vi "dV(dRo)Arch.vi"() -> ()   [LabVIEW 2023]
panel:
  out "x > y?":bool
  out "L см":dbl format="%#_3f"
  out "v м3":dbl format="%#_3f"
  out "Enum":enum16{"ХОВ", "Бор"}(ring)
  in  "dRo":dbl
  in  "N ГЦП":dbl
  in  "C подпитка":dbl
  in  "C крайно":dbl
  in  "C начално":dbl
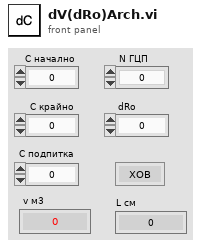
[diagram p1: front panel]
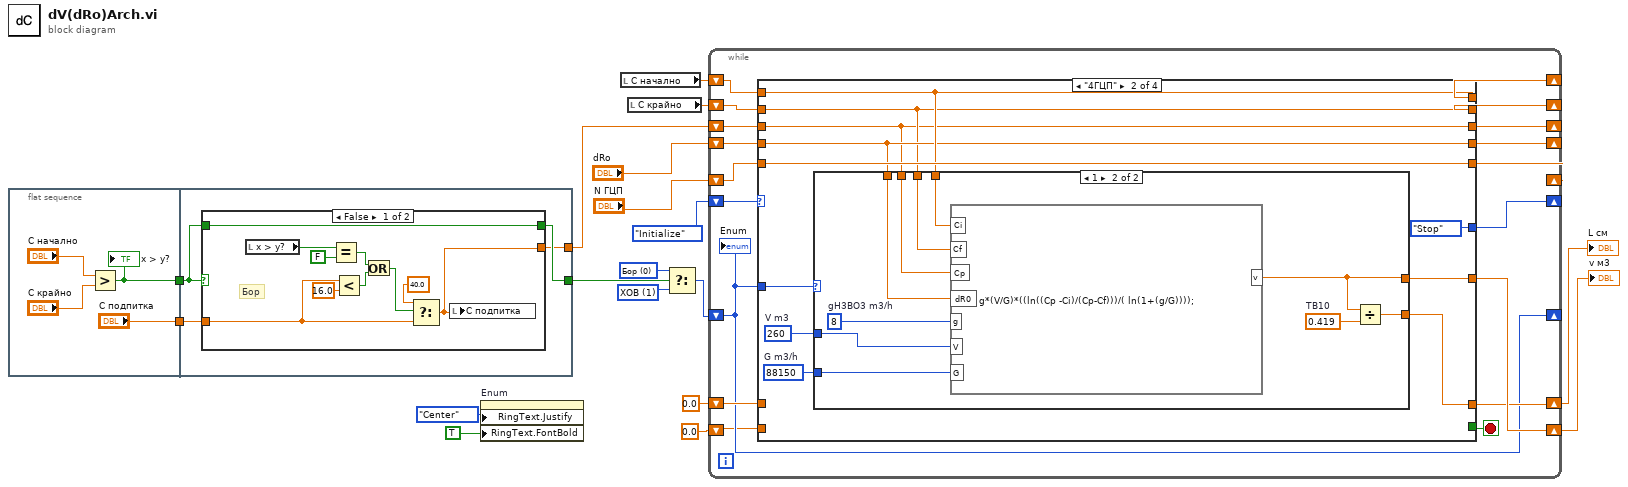
[diagram p0: block diagram]
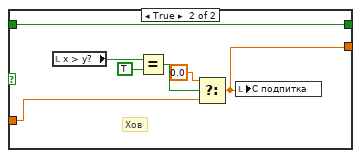
[diagram p2: hidden frame]
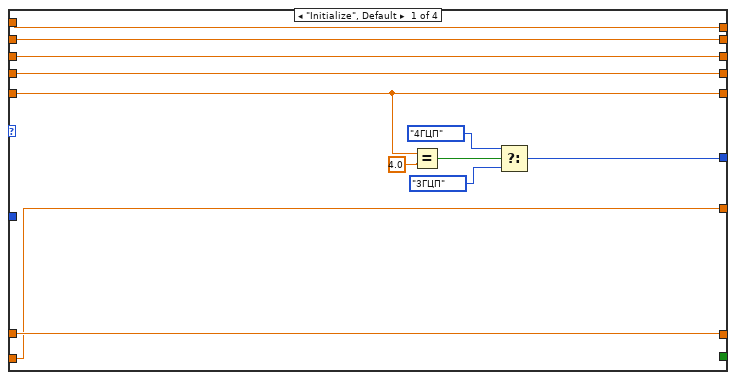
[diagram p3: hidden frame]
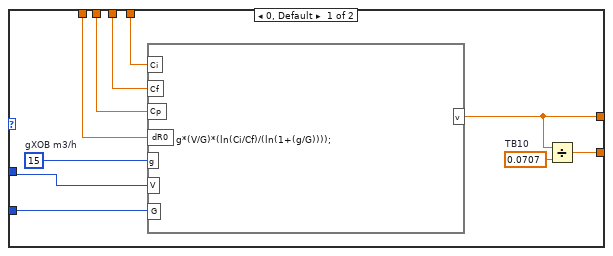
[diagram p4: hidden frame]
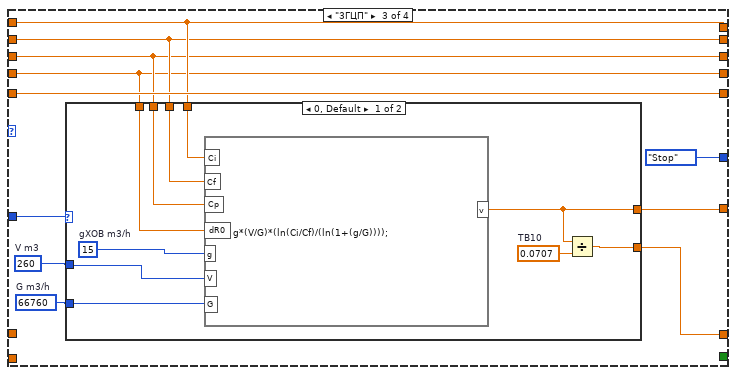
[diagram p5: hidden frame]
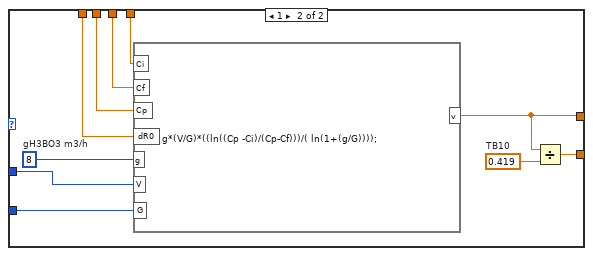
[diagram p6: hidden frame]
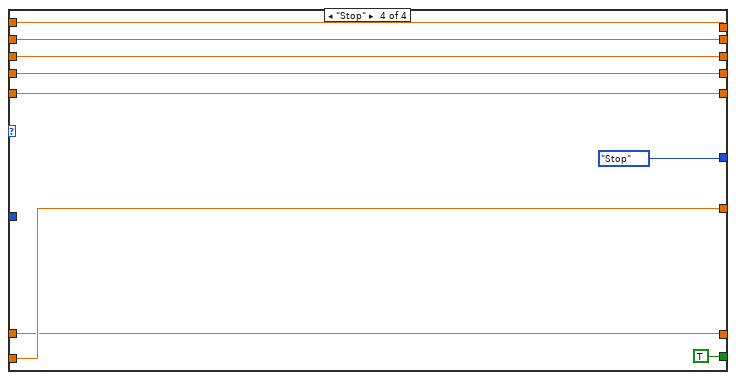
[diagram p7: hidden frame]
diagram:
  w12 = u16 0 items=["Бор", "ХОВ"]
  w13 = u16 1 items=["Бор", "ХОВ"]
  n1 = flat-sequence {
    tunnel: [w22] -> w7
    tunnel: ["C подпитка"] -> w5
    tunnel: [w25] -> w8
    tunnel: w7 -> [w26]
    tunnel: [w24] -> w6
    tunnel: w5 -> [w23]
    frame #0 {
      n2 = Greater?(x="C начално", y="C крайно") -> (0:w22:bool)
      "x > y?" <- w22
    }
    frame #1 {
      n3 = case shown="False" w26 {
        tunnel: w26 -> [w29 w43]
        tunnel: [w29 w43] -> w25
        tunnel: [w28 w37] -> w24
        tunnel: w23 -> [w27 w38]
        frame False {
          # "Бор"
          n4 = local read "x > y?"() -> (w33:bool)
          n5 = Equal?(x=w33, y=FALSE) -> (x = y?=w35:bool)
          n6 = Less?(x=w27, y=16.0) -> (x < y?=w34:bool)
          n7 = Or(x=w35, y=w34) -> (x .or. y?=w36:bool)
          n8 = Select(t=40.0, s=w36, f=w27) -> (s? t:f=w28:dbl)
          n9 = local write "C подпитка"(w28) -> ()
        }
        frame True {
          # "Хов"
          n10 = local read "x > y?"() -> (w41:bool)
          n11 = Equal?(x=w41, y=TRUE) -> (x = y?=w42:bool)
          n12 = Select(t=0.0, s=w42, f=w38) -> (s? t:f=w37:dbl)
          n13 = local write "C подпитка"(w37) -> ()
        }
      }
    }
  }
  n14 = property on="Enum" class="Enum (strict)"("RingText.Justify"=enum16{"Left", "Center", "Right"}."Center" ("Ring Text.Justification"), "RingText.FontBold"=TRUE ("Ring Text.Font:Bold")) -> ()  [unwired: 2 in, 2 out]
  n15 = local read "C начално"() -> (w4:dbl)
  n16 = local read "C крайно"() -> (w3:dbl)
  n17 = Select(t=w12, s=w8, f=w13) -> (s? t:f=w14:u16)
  n18 = while {
    shift-right: [w59] -> _
    shift-left: w4 -> [w60]
    shift-right: [w57] -> _
    shift-left: w3 -> [w58]
    shift-right: [w55] -> _
    shift-left: w6 -> [w56]
    shift-right: [w53] -> _
    shift-left: "dRo" -> [w54]
    shift-right: [w50] -> _
    shift-left: enum16{"Initialize", "4ГЦП", "3ГЦП", "Stop"}."Initialize" -> [w61]
    shift-right: [w51] -> _
    shift-left: "N ГЦП" -> [w52]
    shift-right: [w47] -> w9
    shift-left: 0.0 ("v") -> [w46]
    shift-right: [w45] -> _
    shift-left: w14 -> [w45]
    shift-right: [w48] -> w11
    shift-left: 0.0 ("v") -> [w44]
    stop <- w49 stop-if-true
    n19 = case shown="\"4ГЦП\"" w61 {
      tunnel: w60 -> [w73 w81 w114 w143]
      tunnel: [w73 w81 w114 w143] -> w59
      tunnel: w58 -> [w72 w79 w113 w142]
      tunnel: [w72 w79 w113 w142] -> w57
      tunnel: w56 -> [w71 w78 w112 w141]
      tunnel: [w71 w78 w112 w141] -> w55
      tunnel: w54 -> [w62 w80 w111 w140]
      tunnel: [w62 w80 w111 w140] -> w53
      tunnel: w52 -> [w70 w82 w115 w144]
      tunnel: [w70 w82 w115 w144] -> w51
      tunnel: [w65 enum16{"Initialize", "4ГЦП", "3ГЦП", "Stop"}."Stop" enum16{"Initialize", "4ГЦП", "3ГЦП", "Stop"}."Stop" enum16{"Initialize", "4ГЦП", "3ГЦП", "Stop"}."Stop"] -> w50
      tunnel: [w63 w75 w106 w137] -> w48
      tunnel: [_ _ _ TRUE] -> w49
      tunnel: [w64 w74 w105 w136] -> w47
      tunnel: w46 -> [w64 _ _ w136]
      tunnel: w45 -> [_ w76 w107 _]
      tunnel: w44 -> [w63 _ _ w137]
      frame "Initialize", Default {
        n20 = Equal?(x=w70, y=4.0) -> (x = y?=w68:bool)
        n21 = Select(t=enum16{"Initialize", "4ГЦП", "3ГЦП"}."4ГЦП", s=w68, f=enum16{"Initialize", "4ГЦП", "3ГЦП"}."3ГЦП") -> (s? t:f=w65:enum16{"Initialize", "4ГЦП", "3ГЦП"})
      }
      frame "4ГЦП" {
        w83 = 88150  # G m3/h
        w84 = 260  # V m3
        n22 = case shown="1" w76 {
          tunnel: w84 -> [w93 w101]
          tunnel: w83 -> [w94 w102]
          tunnel: w80 -> [w91 w103]
          tunnel: w78 -> [w90 w96]
          tunnel: w79 -> [w89 w104]
          tunnel: w81 -> [w88 w95]
          tunnel: [w86 w98] -> w75
          tunnel: [w85 w97] -> w74
          frame 0, Default {
            w87 = 0.0707  # TB10
            w92 = 15  # gХОВ m3/h
            n23 = formula code="v = g*(V/G)*(ln(Ci/Cf)/(ln(1+(g/G))));"("Ci"=w88, "Cf"=w89, "Cp"=w90, "dR0"=w91, "g"=w92, "V"=w93, "G"=w94) -> ("v"=w86:dbl)
            n24 = Divide(x=w86, y=w87) -> (x/y=w85:dbl)
          }
          frame 1 {
            w99 = 0.419  # TB10
            w100 = 8  # gH3BO3 m3/h
            n25 = formula code="v = g*(V/G)*((ln((Cp -Ci)/(Cp-Cf)))/( ln(1+(g/G))));"("Ci"=w95, "Cf"=w104, "Cp"=w96, "dR0"=w103, "g"=w100, "V"=w101, "G"=w102) -> ("v"=w98:dbl)
            n26 = Divide(x=w98, y=w99) -> (x/y=w97:dbl)
          }
        }
      }
      frame "3ГЦП" {
        w110 = 66760  # G m3/h
        w109 = 260  # V m3
        n27 = case shown="0, Default" w107 {
          tunnel: w109 -> [w124 w130]
          tunnel: w110 -> [w125 w131]
          tunnel: w111 -> [w122 w132]
          tunnel: w112 -> [w121 w133]
          tunnel: w113 -> [w120 w134]
          tunnel: w114 -> [w119 w135]
          tunnel: [w117 w126] -> w106
          tunnel: [w116 w127] -> w105
          frame 0, Default {
            w118 = 0.0707  # TB10
            w123 = 15  # gХОВ m3/h
            n28 = formula code="v = g*(V/G)*(ln(Ci/Cf)/(ln(1+(g/G))));"("Ci"=w119, "Cf"=w120, "Cp"=w121, "dR0"=w122, "g"=w123, "V"=w124, "G"=w125) -> ("v"=w117:dbl)
            n29 = Divide(x=w117, y=w118) -> (x/y=w116:dbl)
          }
          frame 1 {
            w128 = 0.419  # TB10
            w129 = 8  # gH3BO3 m3/h
            n30 = formula code="v = g*(V/G)*((ln((Cp -Ci)/(Cp-Cf)))/( ln(1+(g/G))));"("Ci"=w135, "Cf"=w134, "Cp"=w133, "dR0"=w132, "g"=w129, "V"=w130, "G"=w131) -> ("v"=w126:dbl)
            n31 = Divide(x=w126, y=w128) -> (x/y=w127:dbl)
          }
        }
      }
      frame "Stop" {
      }
    }
    "Enum" <- w45
  }
  "v м3" <- w11
  "L см" <- w9
